vi "scaler64_pulse.vi"(6 "PresetValues_Scaler":u32[](array[numeric])=[0, 0, 0, 0, 0, 0, 0, 0, 0, 0, 0, 0, 0, 0, 0, 0, 0, 0, 0, 0, 0, 0, 0, 0, 0, 0, 0, 0, 0, 0, 0, 0, 0, 0, 0, 0, 0, 0, 0, 0, 0, 0, 0, 0, 0, 0, 0, 0, 0, 0, 0, 0, 0, 0, 0, 0, 0, 0, 0, 0, 0, 0, 0, 0], 8 "Pulse_Scaler":bool[](array[boolean])=[FALSE, FALSE, FALSE, FALSE, FALSE, FALSE, FALSE, FALSE, FALSE, FALSE, FALSE, FALSE, FALSE, FALSE, FALSE, FALSE, FALSE, FALSE, FALSE, FALSE, FALSE, FALSE, FALSE, FALSE, FALSE, FALSE, FALSE, FALSE, FALSE, FALSE, FALSE, FALSE, FALSE, FALSE, FALSE, FALSE, FALSE, FALSE, FALSE, FALSE, FALSE, FALSE, FALSE, FALSE, FALSE, FALSE, FALSE, FALSE, FALSE, FALSE, FALSE, FALSE, FALSE, FALSE, FALSE, FALSE, FALSE, FALSE, FALSE, FALSE, FALSE, FALSE, FALSE, FALSE], 9 "OneShot_Scaler":bool, 10 "Gate_Scaler":bool[](array[boolean])=[FALSE, FALSE, FALSE, FALSE, FALSE, FALSE, FALSE, FALSE, FALSE, FALSE, FALSE, FALSE, FALSE, FALSE, FALSE, FALSE, FALSE, FALSE, FALSE, FALSE, FALSE, FALSE, FALSE, FALSE, FALSE, FALSE, FALSE, FALSE, FALSE, FALSE, FALSE, FALSE, FALSE, FALSE, FALSE, FALSE, FALSE, FALSE, FALSE, FALSE, FALSE, FALSE, FALSE, FALSE, FALSE, FALSE, FALSE, FALSE, FALSE, FALSE, FALSE, FALSE, FALSE, FALSE, FALSE, FALSE, FALSE, FALSE, FALSE, FALSE, FALSE, FALSE, FALSE, FALSE], 11 "Enable_Scaler":bool) -> (2 "Counter_Scaler":u32[](array[numeric]), 3 "Done_Scaler":bool)   [LabVIEW 2017]
uses:
  <vilib>/rvi/IPIntegrationNode/IPINode_Typedef/niFpgaIPINodeSupportedFamilies.ctl
  <vilib>/rvi/IPIntegrationNode/IPINode_Utilities/niFpgaIPINodeSimCore.vi
  <vilib>/rvi/IPIntegrationNode/IPINode_Xnode/niFpgaIPINode.xnode
  scaler_vhdl/src/Scaler64_5SimFiles/xsim.dir/scaler_64_lv_wrapper/xsimkE7343CD01BD446888FE8A1ECD56163F1.dll
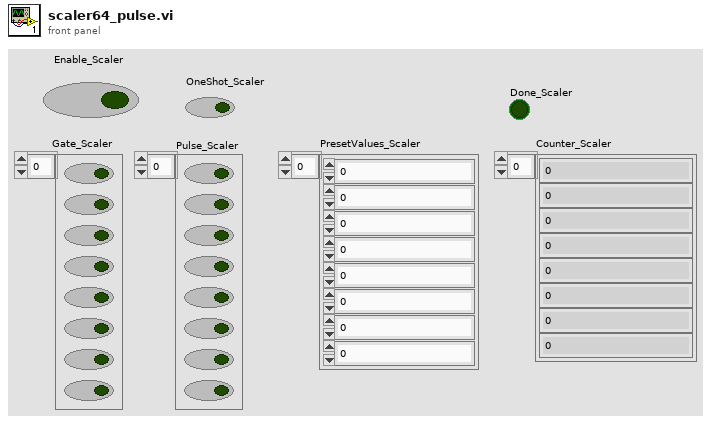
[diagram p1: front panel]
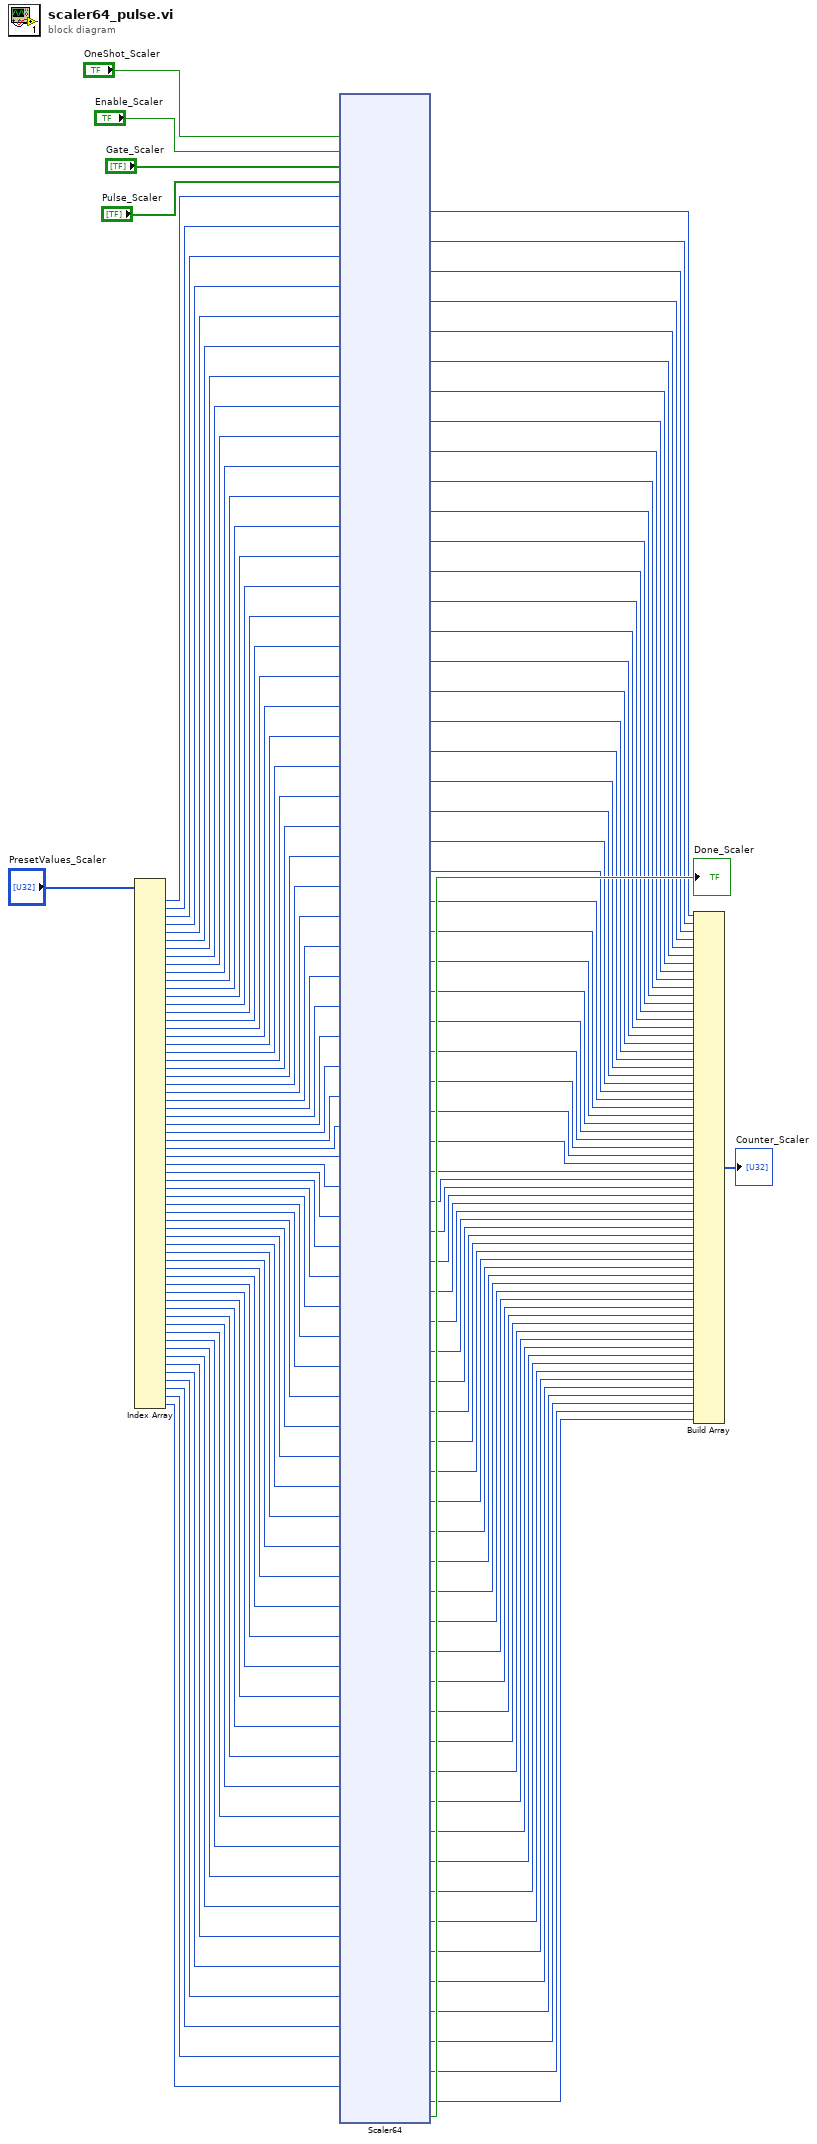
[diagram p0: block diagram]
diagram:
  n1 = Index Array(array="PresetValues_Scaler") -> (element #1=w131:u32, element #2=w130:u32, element #3=w129:u32, element #4=w128:u32, element #5=w127:u32, element #6=w126:u32, element #7=w125:u32, element #8=w124:u32, element #9=w123:u32, element #10=w122:u32, element #11=w121:u32, element #12=w120:u32, element #13=w119:u32, element #14=w118:u32, element #15=w117:u32, element #16=w116:u32, element #17=w115:u32, element #18=w114:u32, element #19=w113:u32, element #20=w112:u32, element #21=w111:u32, element #22=w110:u32, element #23=w109:u32, element #24=w108:u32, element #25=w107:u32, element #26=w106:u32, element #27=w105:u32, element #28=w104:u32, element #29=w103:u32, element #30=w102:u32, element #31=w101:u32, element #32=w100:u32, element #33=w99:u32, element #34=w98:u32, element #35=w97:u32, element #36=w96:u32, element #37=w95:u32, element #38=w94:u32, element #39=w93:u32, element #40=w92:u32, element #41=w91:u32, element #42=w90:u32, element #43=w89:u32, element #44=w88:u32, element #45=w87:u32, element #46=w86:u32, element #47=w85:u32, element #48=w84:u32, element #49=w83:u32, element #50=w82:u32, element #51=w81:u32, element #52=w80:u32, element #53=w79:u32, element #54=w78:u32, element #55=w77:u32, element #56=w76:u32, element #57=w75:u32, element #58=w74:u32, element #59=w73:u32, element #60=w72:u32, element #61=w71:u32, element #62=w70:u32, element #63=w69:u32, element #64=w68:u32)  [unwired: 64 in]
  n2 = xnode ("Scaler64")("one_shot_i"="OneShot_Scaler", "scaler_enable_i"="Enable_Scaler", "gate_i"="Gate_Scaler", "pulse_i"="Pulse_Scaler", "preset_value_0_i"=w131, "preset_value_1_i"=w130, "preset_value_2_i"=w129, "preset_value_3_i"=w128, "preset_value_4_i"=w127, "preset_value_5_i"=w126, "preset_value_6_i"=w125, "preset_value_7_i"=w124, "preset_value_8_i"=w123, "preset_value_9_i"=w122, "preset_value_10_i"=w121, "preset_value_11_i"=w120, "preset_value_12_i"=w119, "preset_value_13_i"=w118, "preset_value_14_i"=w117, "preset_value_15_i"=w116, "preset_value_16_i"=w115, "preset_value_17_i"=w114, "preset_value_18_i"=w113, "preset_value_19_i"=w112, "preset_value_20_i"=w111, "preset_value_21_i"=w110, "preset_value_22_i"=w109, "preset_value_23_i"=w108, "preset_value_24_i"=w107, "preset_value_25_i"=w106, "preset_value_26_i"=w105, "preset_value_27_i"=w104, "preset_value_28_i"=w103, "preset_value_29_i"=w102, "preset_value_30_i"=w101, "preset_value_31_i"=w100, "preset_value_32_i"=w99, "preset_value_33_i"=w98, "preset_value_34_i"=w97, "preset_value_35_i"=w96, "preset_value_36_i"=w95, "preset_value_37_i"=w94, "preset_value_38_i"=w93, "preset_value_39_i"=w92, "preset_value_40_i"=w91, "preset_value_41_i"=w90, "preset_value_42_i"=w89, "preset_value_43_i"=w88, "preset_value_44_i"=w87, "preset_value_45_i"=w86, "preset_value_46_i"=w85, "preset_value_47_i"=w84, "preset_value_48_i"=w83, "preset_value_49_i"=w82, "preset_value_50_i"=w81, "preset_value_51_i"=w80, "preset_value_52_i"=w79, "preset_value_53_i"=w78, "preset_value_54_i"=w77, "preset_value_55_i"=w76, "preset_value_56_i"=w75, "preset_value_57_i"=w74, "preset_value_58_i"=w73, "preset_value_59_i"=w72, "preset_value_60_i"=w71, "preset_value_61_i"=w70, "preset_value_62_i"=w69, "preset_value_63_i"=w68) -> ("counter_0_o"=w66:u32, "counter_1_o"=w65:u32, "counter_2_o"=w64:u32, "counter_3_o"=w63:u32, "counter_4_o"=w62:u32, "counter_5_o"=w61:u32, "counter_6_o"=w60:u32, "counter_7_o"=w59:u32, "counter_8_o"=w58:u32, "counter_9_o"=w57:u32, "counter_10_o"=w56:u32, "counter_11_o"=w55:u32, "counter_12_o"=w54:u32, "counter_13_o"=w53:u32, "counter_14_o"=w52:u32, "counter_15_o"=w51:u32, "counter_16_o"=w50:u32, "counter_17_o"=w49:u32, "counter_18_o"=w48:u32, "counter_19_o"=w47:u32, "counter_20_o"=w46:u32, "counter_21_o"=w45:u32, "counter_22_o"=w44:u32, "counter_23_o"=w43:u32, "counter_24_o"=w42:u32, "counter_25_o"=w41:u32, "counter_26_o"=w40:u32, "counter_27_o"=w39:u32, "counter_28_o"=w38:u32, "counter_29_o"=w37:u32, "counter_30_o"=w36:u32, "counter_31_o"=w35:u32, "counter_32_o"=w34:u32, "counter_33_o"=w33:u32, "counter_34_o"=w32:u32, "counter_35_o"=w31:u32, "counter_36_o"=w30:u32, "counter_37_o"=w29:u32, "counter_38_o"=w28:u32, "counter_39_o"=w27:u32, "counter_40_o"=w26:u32, "counter_41_o"=w25:u32, "counter_42_o"=w24:u32, "counter_43_o"=w23:u32, "counter_44_o"=w22:u32, "counter_45_o"=w21:u32, "counter_46_o"=w20:u32, "counter_47_o"=w19:u32, "counter_48_o"=w18:u32, "counter_49_o"=w17:u32, "counter_50_o"=w16:u32, "counter_51_o"=w15:u32, "counter_52_o"=w14:u32, "counter_53_o"=w13:u32, "counter_54_o"=w12:u32, "counter_55_o"=w11:u32, "counter_56_o"=w10:u32, "counter_57_o"=w9:u32, "counter_58_o"=w8:u32, "counter_59_o"=w7:u32, "counter_60_o"=w6:u32, "counter_61_o"=w5:u32, "counter_62_o"=w4:u32, "counter_63_o"=w3:u32, "done_o"=→"Done_Scaler":bool)  [unwired: 2 in]
  n3 = Build Array(w66, w65, w64, w63, w62, w61, w60, w59, w58, w57, w56, w55, w54, w53, w52, w51, w50, w49, w48, w47, w46, w45, w44, w43, w42, w41, w40, w39, w38, w37, w36, w35, w34, w33, w32, w31, w30, w29, w28, w27, w26, w25, w24, w23, w22, w21, w20, w19, w18, w17, w16, w15, w14, w13, w12, w11, w10, w9, w8, w7, w6, w5, w4, w3) -> (→"Counter_Scaler":u32[])
